vi "Set Power.vi"(8 "error in (no error)":errorcluster, 10 "Power":i32 min=0 max=5 step=1, 11 "Julabo FP-50 Settings":T1={"VISA resource name"="", "Simulated?"=FALSE, "Pump Power"=2} {"Pump Power" min=0 max=8 step=1}) -> (0 "error out":errorcluster, 1 "Connection Error":bool, 3 "Julabo FP-50 Settings":T1={"VISA resource name"="", "Simulated?"=FALSE, "Pump Power"=2} {"Pump Power" min=0 max=8 step=1})   [LabVIEW 2018, in "Julabo Type FP-50 TCU.lvlib"]
uses:
  Julabo Type FP-50 TCU.lvlib
  Julabo FP-50 Settings.ctl
  Third Party Drivers/Julabo Type 1/JULABO DeviceDriver/JULABO DeviceDriver.lvlib
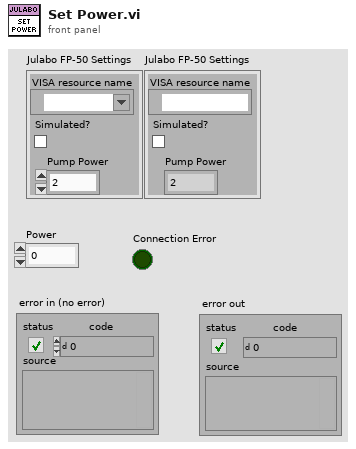
[diagram p1: front panel]
types:
  T1 = typedef "Julabo Type FP-50 TCU.lvlib/Julabo FP-50 Settings.ctl" = cluster{"VISA resource name":refnum<visa-resource-name>, "Simulated?":bool, "Pump Power":i32}
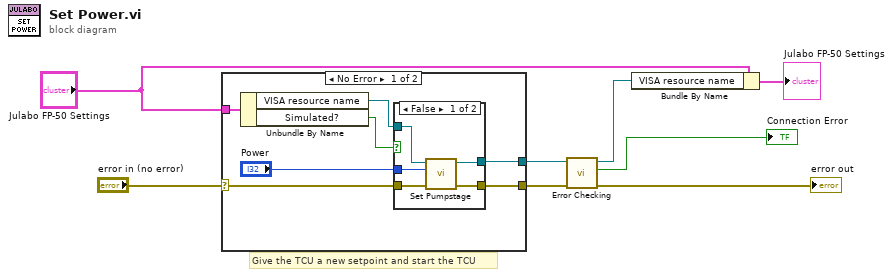
[diagram p0: block diagram]
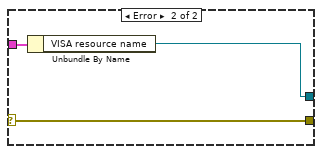
[diagram p3: hidden frame]
diagram:
  # "Give the TCU a new setpoint and start the TCU"
  n1 = case shown="No Error" "error in (no error)" {
    selector: "error in (no error)" -> [w15 w25]
    tunnel: "Julabo FP-50 Settings" -> [w11 w24]
    tunnel: [w14 w25] -> w6
    tunnel: [w13 w23] -> w7
    frame No Error {
      n2 = Unbundle By Name(w11) -> ("VISA resource name"=w9:refnum<visa-resource-name>, "Simulated?"=w12:bool)
      n3 = case shown="False" w12 {
        tunnel: w15 -> [w17 w22]
        tunnel: [w16 w22] -> w14
        tunnel: [w19 w21] -> w13
        tunnel: w9 -> [w20 w21]
        tunnel: "Power" -> [w18 _]
        frame False {
          n4 = call "Set Pumpstage.vi"("error in (no error)"=w17, "Pumpstage (1: default)"=w18, "VISA resource name"=w20) -> ("error out"=w16:errorcluster, "VISA resource name out"=w19:refnum<visa-resource-name>)  [unwired: 7 in]
        }
        frame True {
        }
      }
    }
    frame Error {
      n5 = Unbundle By Name(w24) -> ("VISA resource name"=w23:refnum<visa-resource-name>)
    }
  }
  n6 = call "Error Checking.vi"("error in (no error)"=w6, "VISA resource name"=w7) -> ("error out"=→"error out":errorcluster, "Connection Error"=→"Connection Error":bool, "VISA resource name"=w4:refnum<visa-resource-name>)  [unwired: 7 in]
  n7 = Bundle By Name(cluster="Julabo FP-50 Settings", "VISA resource name"=w4) -> (→"Julabo FP-50 Settings":T1)
